vi "Write Keepalive.vi"(8 "error in (no error)":errorcluster, 10 "Keepalive":T1={"Enabled"=FALSE, "Ping Interval (ms)"=25000, "Ping Timeout (ms)"=20000}, 11 "Keepalive Heartbeat in":refnum<class "Keepalive Heartbeat.lvclass">) -> (0 "error out":errorcluster, 3 "Keepalive Heartbeat out":refnum<class "Keepalive Heartbeat.lvclass">)   [LabVIEW 2021, in "WebSocket Actors.lvlib" / "Keepalive Heartbeat.lvclass"]
uses:
  Keepalive Heartbeat.lvclass
  WebSocket Connection/Keepalive.ctl
  Keepalive Heartbeat.lvclass/Keepalive Heartbeat.ctl
  WebSocket Connection/WebSocket Connection.lvclass
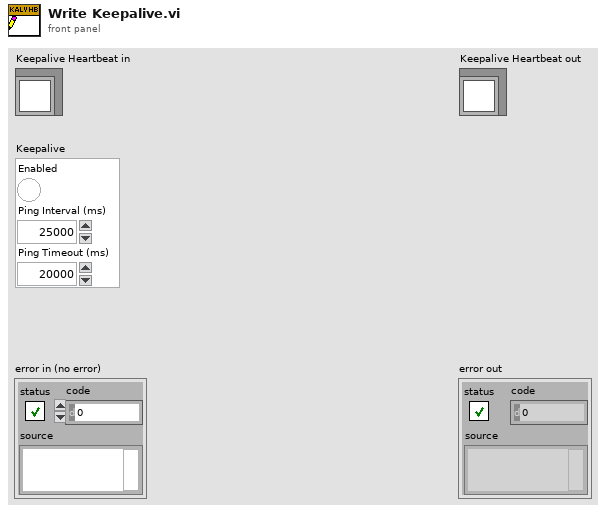
[diagram p1: front panel]
types:
  T1 = typedef "WebSocket Actors.lvlib/WebSocket Connection.lvclass/Keepalive.ctl" = cluster{"Enabled":bool, "Ping Interval (ms)":u32, "Ping Timeout (ms)":u32}
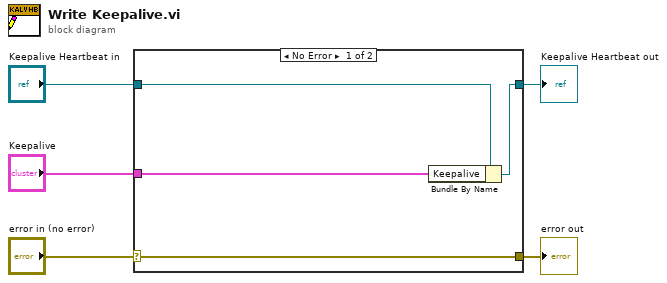
[diagram p0: block diagram]
diagram:
  n1 = case shown="No Error" "error in (no error)" {
    selector: "error in (no error)" -> [w9 w10]
    tunnel: [w9 w10] -> w4
    tunnel: [w7 w11] -> w2
    tunnel: "Keepalive Heartbeat in" -> [w8 w11]
    tunnel: "Keepalive" -> [w6 _]
    frame No Error {
      n2 = Bundle By Name(cluster=w8, "Keepalive"=w6) -> (w7:refnum<class "Keepalive Heartbeat.lvclass">)
    }
    frame Error {
    }
  }
  "error out" <- w4
  "Keepalive Heartbeat out" <- w2
